vi "ReadConfigFile.vi"(8 "error in (no error)":errorcluster, 11 "Microscope in":refnum<class "Microscope.lvclass">) -> (0 "error out":errorcluster, 3 "Microscope out":refnum<class "Microscope.lvclass">)   [LabVIEW 2020, in "Microscope.lvlib" / "Microscope.lvclass"]
uses:
  Microscope.lvclass
  Microscope.lvclass/Microscope.ctl
  Component/Device/Device/Device.lvclass
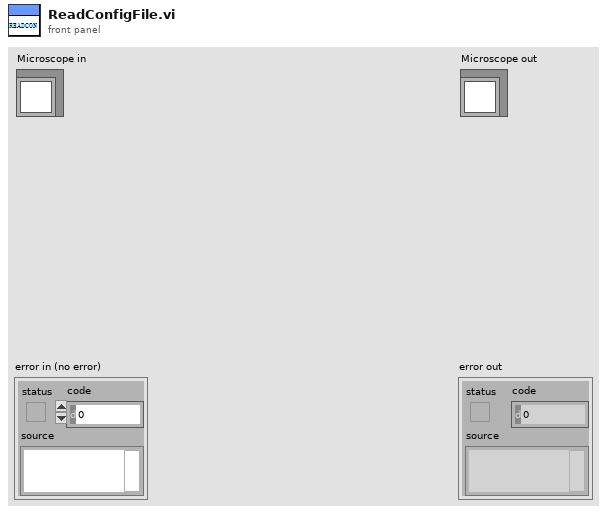
[diagram p1: front panel]
types:
  T1 = cluster{"Values[0]":i32, "Values[1]":i32, "Values[2]":i32}
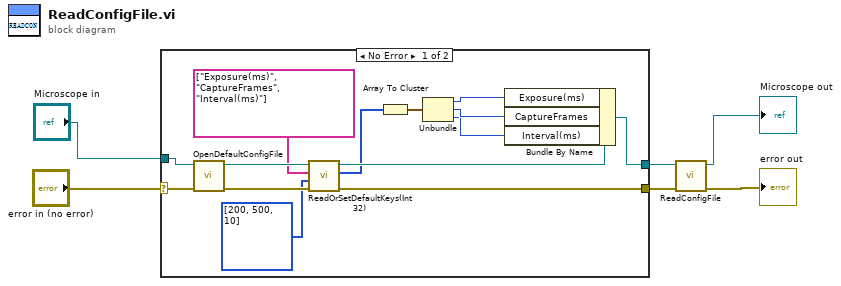
[diagram p0: block diagram]
diagram:
  n1 = case shown="No Error" "error in (no error)" {
    selector: "error in (no error)" -> [w20 w21]
    tunnel: [w17 w21] -> w4
    tunnel: [w13 w22] -> w2
    tunnel: "Microscope in" -> [w19 w22]
    frame No Error {
      n2 = call-dynamic "OpenDefaultConfigFile.vi"("error in (no error)"=w20, "Device in"=w19) -> ("error out"=w18:errorcluster, "Device out"=w16:refnum<class "Microscope.lvclass">)  [unwired: 7 in, 1 out]
      n3 = call-dynamic "ReadOrSetDefaultKeys(Int32).vi"("error in (no error)"=w18, "Default"=i32[] [200, 500, 10], "Keys"=string[] ["Exposure(ms)", "CaptureFrames", "Interval(ms)"], "Device in"=w16) -> ("error out"=w17:errorcluster, "Values"=w12:i32[], "Device out"=w15:refnum<class "Microscope.lvclass">)  [unwired: 5 in]
      n4 = Array To Cluster(array=w12) -> (cluster=w11:T1)
      n5 = Unbundle(w11) -> ("Values[0]"=w10:i32, "Values[1]"=w9:i32, "Values[2]"=w8:i32)
      n6 = Bundle By Name(cluster=w15, "Exposure(ms)"=w10, "CaptureFrames"=w9, "Interval(ms)"=w8) -> (w13:refnum<class "Microscope.lvclass">)
    }
    frame Error {
    }
  }
  n7 = call-parent "ReadConfigFile.vi"("error in (no error)"=w4, "Device in"=w2) -> ("error out"=→"error out":errorcluster, "Device out"=→"Microscope out":refnum<class "Microscope.lvclass">)  [unwired: 8 in]
